vi "Helmholtz2D_FEM_Inpolygon_Intersect.vi"(8 "x":cdb, 9 "next x":cdb, 10 "p":cdb, 11 "p+dp":cdb) -> (2 "mu":dbl, 3 "lambda":dbl)   [LabVIEW 2017, in "NI_PDE.lvlib"]
uses:
  <vilib>/gmath/NI_PDE.lvlib
  <vilib>/Analysis/7linalg.llb/Solve Linear Equations (single right hand).vi
  <vilib>/Analysis/baseanly.llb/Solve Linear Equations By Cholesky.vi
  <vilib>/Analysis/baseanly.llb/Real Matrix to Compact Array.vi
  <vilib>/Analysis/baseanly.llb/Real Compact Tri-Matrix Linear Eqs.vi
  <vilib>/Analysis/7linalg.llb/Solve Linear Eqs (General).vi
  <vilib>/Analysis/7linalg.llb/Solve Linear Eqs (Gen, single right hand).vi
  <vilib>/Analysis/NI_AALPro.lvlib
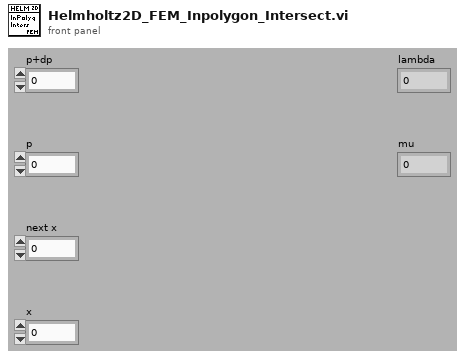
[diagram p1: front panel]
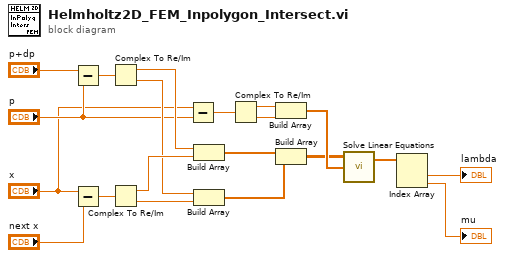
[diagram p0: block diagram]
diagram:
  n1 = Subtract(x="p+dp", y="p") -> (x-y=w20:cdb)
  n2 = Subtract(x="x", y="next x") -> (x-y=w19:cdb)
  n3 = Complex To Re/Im(x + iy=w20) -> (x=w18:dbl, y=w16:dbl)
  n4 = Complex To Re/Im(x + iy=w19) -> (x=w17:dbl, y=w15:dbl)
  n5 = Subtract(x="x", y="p") -> (x-y=w12:cdb)
  n6 = Build Array(w18, w17) -> (w14:dbl[])
  n7 = Build Array(w16, w15) -> (w13:dbl[])
  n8 = Complex To Re/Im(x + iy=w12) -> (x=w11:dbl, y=w10:dbl)
  n9 = Build Array(w11, w10) -> (w9:dbl[])
  n10 = Build Array(w14, w13) -> (w7:dbl[][])
  n11 = call-poly <vilib>:"Solve Linear Equations.vi"("Known Vector"=w9, "Input Matrix"=w7) -> ("Solution Vector"=w8:dbl[])  [unwired: 1 in, 1 out]
  n12 = Index Array(array=w8) -> (element #1=→"lambda":dbl, element #2=→"mu":dbl)  [unwired: 2 in]
